vi "Begin.vi"(8 "error in":errorcluster) -> (0 "error out":errorcluster)   [LabVIEW 2015]
doc: "Called before other user functions, this VI is expected to open initial I/O refnums, load in file data, and do all program initialization. Notice that the <B>error out</B> terminal is simply used for data flow. Wiring it to other structures or subVIs ensures that this VI runs first."
uses:
  <vilib>/Rock Robotics/WPI/DriverStation/WPI_DriverStationRobotMode2.ctl
  <vilib>/Rock Robotics/WPI/Joystick/WPI_JoystickDeviceEnum.ctl
  <vilib>/Rock Robotics/SystemInterfaces/spilib/spi_bus.ctl
  <vilib>/Rock Robotics/WPI/CAN/TalonSRX/WPI_CANTalonSRX_APIControlMode.ctl
  <vilib>/Rock Robotics/WPI/CAN/TalonSRX/WPI_CANTalonSRX_APIFeedbackSelect.ctl
  <vilib>/Rock Robotics/SystemInterfaces/DIO/FPGA_DIOPWMChannel.ctl
  <vilib>/Rock Robotics/WPI/Solenoid/WPI_SolenoidChannel.ctl
  Robot Global Data.vi
  <vilib>/Rock Robotics/WPI/MotorControl/WPI_MotorControlOpenCANTalonSRX.vi
  <vilib>/Rock Robotics/WPI/Gyro/WPI_GyroXRS450_SPI_Open.vi
  <vilib>/Rock Robotics/WPI/Utilities/WPI_GetSetVariantRefNum.vi
  <vilib>/Rock Robotics/WPI/MotorControl/WPI_MotorControlOpen Talon.vi
  <vilib>/Rock Robotics/WPI/Solenoid/WPI_SolenoidOpenSingle.vi
  <vilib>/Rock Robotics/WPI/Solenoid/WPI_SolenoidOpenDouble.vi
  <vilib>/Rock Robotics/WPI/Counter/WPI_CounterDigitalInputToDigitalSource.vi
  <vilib>/Rock Robotics/SystemInterfaces/DIO/FPGA_DIOChannel.ctl
  <vilib>/Rock Robotics/WPI/Encoder/WPI_EncoderType.ctl
  <vilib>/Rock Robotics/SystemInterfaces/AI/FPGA_AIChannel.ctl
  <vilib>/Rock Robotics/WPI/Ultrasonic/WPI_SonarMB1010AnalogRefNum Registry Set.vi
  <vilib>/Rock Robotics/WPI/Ultrasonic/WPI_SonarMB1010AnalogOpen.vi
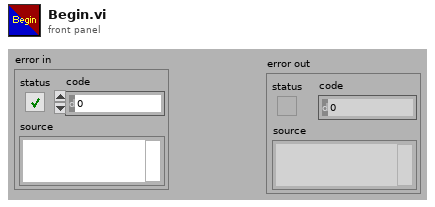
[diagram p1: front panel]
types:
  T1 = typedef "WPI_CANTalonSRX_APIFeedbackSelect.ctl" = enum16{"Digital Quadrature Encoder", "Analog Potentiometer", "Analog Encoder", "Count on Quad-A (Rising-Edge)", "Count on Quad-A (Falling-Edge)", "CTR Magnetic Enc (Absolute)", "CTR Magnetic Enc (Relative)", "Pulse Width"}
  T2 = typedef "FPGA_DIOPWMChannel.ctl" = enum8{"PWM 0", "PWM 1", "PWM 2", "PWM 3", "PWM 4", "PWM 5", "PWM 6", "PWM 7", "PWM 8", "PWM 9", "PWM MXP 0", "PWM MXP 1", "PWM MXP 2", "PWM MXP 3", "PWM MXP 4", "PWM MXP 5", "PWM MXP 6", "PWM MXP 7", "PWM MXP 8", "PWM MXP 9", "Invalid"}
  T3 = typedef "WPI_JoystickDeviceEnum.ctl" = enum16{"USB 0", "USB 1", "USB 2", "USB 3", "USB 4", "USB 5"}
  T4 = typedef "WPI_CANTalonSRX_APIControlMode.ctl" = enum8{"Percent VBus", "Speed", "Position", "Slave", "Unchanged / Invalid", "Voltage Compensation", "Current", "Motion Profile"}
  T5 = typedef "spi_bus.ctl" = enum16{"SPI On-Board, CS0", "SPI On-Board, CS1", "SPI On-Board, CS2", "SPI On-Board, CS3", "SPI MXP", "Invalid"}
  T6 = typedef "WPI_DriverStationRobotMode2.ctl" = enum16{"Autonomous Disabled", "Autonomous Enabled", "Teleop Disabled", "Teleop Enabled", "Disconnected", "Finish", "Test Disabled", "Test Enabled", "Emergency Stopped"}
  T7 = typedef "FPGA_AIChannel.ctl" = enum8{"AI 0", "AI 1", "AI 2", "AI 3", "AI MXP 0", "AI MXP 1", "AI MXP 2", "AI MXP 3", "Invalid"}
  T8 = typedef "WPI_SonarMB1010AnalogDeviceRef.ctl" = cluster{"AIDeviceRef":T9, "Scaling factor (V/in)":dbl, "Average Bits":u8}
  T9 = typedef "WPI_AnalogChannelDevRef.ctl" = cluster{"DevStatus":errorcluster, "Analog Channel":T7}
  T10 = typedef "WPI_SolenoidChannel.ctl" = enum8{"Solenoid 0", "Solenoid 1", "Solenoid 2", "Solenoid 3", "Solenoid 4", "Solenoid 5", "Solenoid 6", "Solenoid 7", "Invalid"}
  T11 = typedef "WPI_ServoDeviceRef.ctl" = cluster{"DeviceStatus":errorcluster, "PWM Channel":T2, "DeadBand":T12}
  T12 = typedef "WPI_PWMDeadband.ctl" = cluster{"Name":string, "maxPositivePwm":i32, "minPositivePwm":i32, "centerPwm":i32, "maxNegativePwm":i32, "minNegativePwm":i32, "angularRange":u16}
  T13 = typedef "WPI_SolenoidDevRef.ctl" = cluster{"DevStatus":errorcluster, "Pneumatics Control Module":u8, "Forward Solenoid Channel":T10, "Reverse Solenoid Channel":T10}
  T14 = typedef "WPI_MotorControlDeviceRef.ctl" = cluster{"DeviceStatus":errorcluster, "Type":T15, "PWM":cluster{"PWM Channel":T2, "DeadBand":T12}, "CAN":cluster{"Device Number":u8, "Control Mode":T16, "Semaphore":T17, "Max Vout":dbl, "TalonSRX Control Mode":T4}, "Invert":bool}
  T15 = typedef "WPI_MotorControlType.ctl" = enum16{"PWM", "CAN", "CANTalonSRX"}
  T16 = typedef "WPI_CANJaguar_ControlMode.ctl" = enum8{"Percent VBus", "Current", "Speed", "Position", "Voltage"}
  T17 = typedef "Semaphore RefNum" = refnum<k1>
  T18 = typedef "WPI_JoystickDevRef.ctl" = cluster{"Device":T3}
  T19 = typedef "WPI_GyroDevRef.ctl" = cluster{"DevStatus":errorcluster, "Analog Channel":T7, "Offset":dbl, "Gain (VoltsPerDegree/Second)":dbl, "Gyro Type":enum16{"Analog", "XRS450"}, "Handle":i32, "SPI Bus":T5, "Device Found":bool, "Sample Rate":dbl, "Calibrate On Open":bool}
  T20 = typedef "WPI_PotentiometerDevRef.ctl" = cluster{"DevStatus":errorcluster, "Analog Channel":T7, "Invert Output":bool}
  T21 = typedef "WPI_CompressorDevRef.ctl" = cluster{"DevStatus":errorcluster, "Pneumatics Control Module":u8}
  T22 = typedef "WPI_EncoderType.ctl" = enum16{"1x", "2x", "4x"}
  T23 = typedef "FPGA_DIOChannel.ctl" = enum8{"DIO 0", "DIO 1", "DIO 2", "DIO 3", "DIO 4", "DIO 5", "DIO 6", "DIO 7", "DIO 8", "DIO 9", "DIO MXP 0", "DIO MXP 1", "DIO MXP 2", "DIO MXP 3", "DIO MXP 4", "DIO MXP 5", "DIO MXP 6", "DIO MXP 7", "DIO MXP 8", "DIO MXP 9", "DIO MXP 10", "DIO MXP 11", "DIO MXP 12", "DIO MXP 13", "DIO MXP 14", "DIO MXP 15", "Invalid"}
  T24 = typedef "WPI_DigitalInputDevRef.ctl" = cluster{"DevStatus":errorcluster, "DIO Channel":T23}
  T25 = typedef "FPGA_CounterEncoderSourceConvertionLVSourceType.ctl" = cluster{"DevStatus":errorcluster, "AnalogTriggerMode?":bool, "DigitalMode":cluster{"DIO Channel":T26}, "AnalogTriggerMode":cluster{"AnalogTriggerIndex":T27, "OutputType":T28}}
  T26 = typedef "FPGA_DIODigitalSourceChannel.ctl" = enum8{"DIO 0", "DIO 1", "DIO 2", "DIO 3", "DIO 4", "DIO 5", "DIO 6", "DIO 7", "DIO 8", "DIO 9", "DIO MXP 0", "DIO MXP 1", "DIO MXP 2", "DIO MXP 3", "DIO MXP 4", "DIO MXP 5", "DIO MXP 6", "DIO MXP 7", "DIO MXP 8", "DIO MXP 9", "DIO MXP 10", "DIO MXP 11", "DIO MXP 12", "DIO MXP 13", "DIO MXP 14", "DIO MXP 15", "Disabled"}
  T27 = typedef "FPGA_AnalogTriggerIndex.ctl" = enum8{"Trig 0", "Trig 1", "Trig 2", "Trig 3", "Trig 4", "Trig 5", "Trig 6", "Trig 7", "Invalid"}
  T28 = typedef "FPGA_AnalogTriggerOutType.ctl" = enum16{"InWindow", "TriggerState", "Rising", "Falling"}
  T29 = typedef "WPI_EncoderDevRef.ctl" = cluster{"DevStatus":errorcluster, "EncoderIndex":T30, "CounterIndex":T31, "DistancePerCount":dbl, "Decoding Type":T22}
  T30 = typedef "FPGA_EncoderIdx.ctl" = enum8{"Enc 0", "Enc 1", "Enc 2", "Enc 3", "Enc 4", "Enc 5", "Enc 6", "Enc 7", "Invalid"}
  T31 = typedef "FPGA_CounterCtrSystemIndex.ctl" = enum8{"Ctr 0", "Ctr 1", "Ctr 2", "Ctr 3", "Ctr 4", "Ctr 5", "Ctr 6", "Ctr 7", "Invalid"}
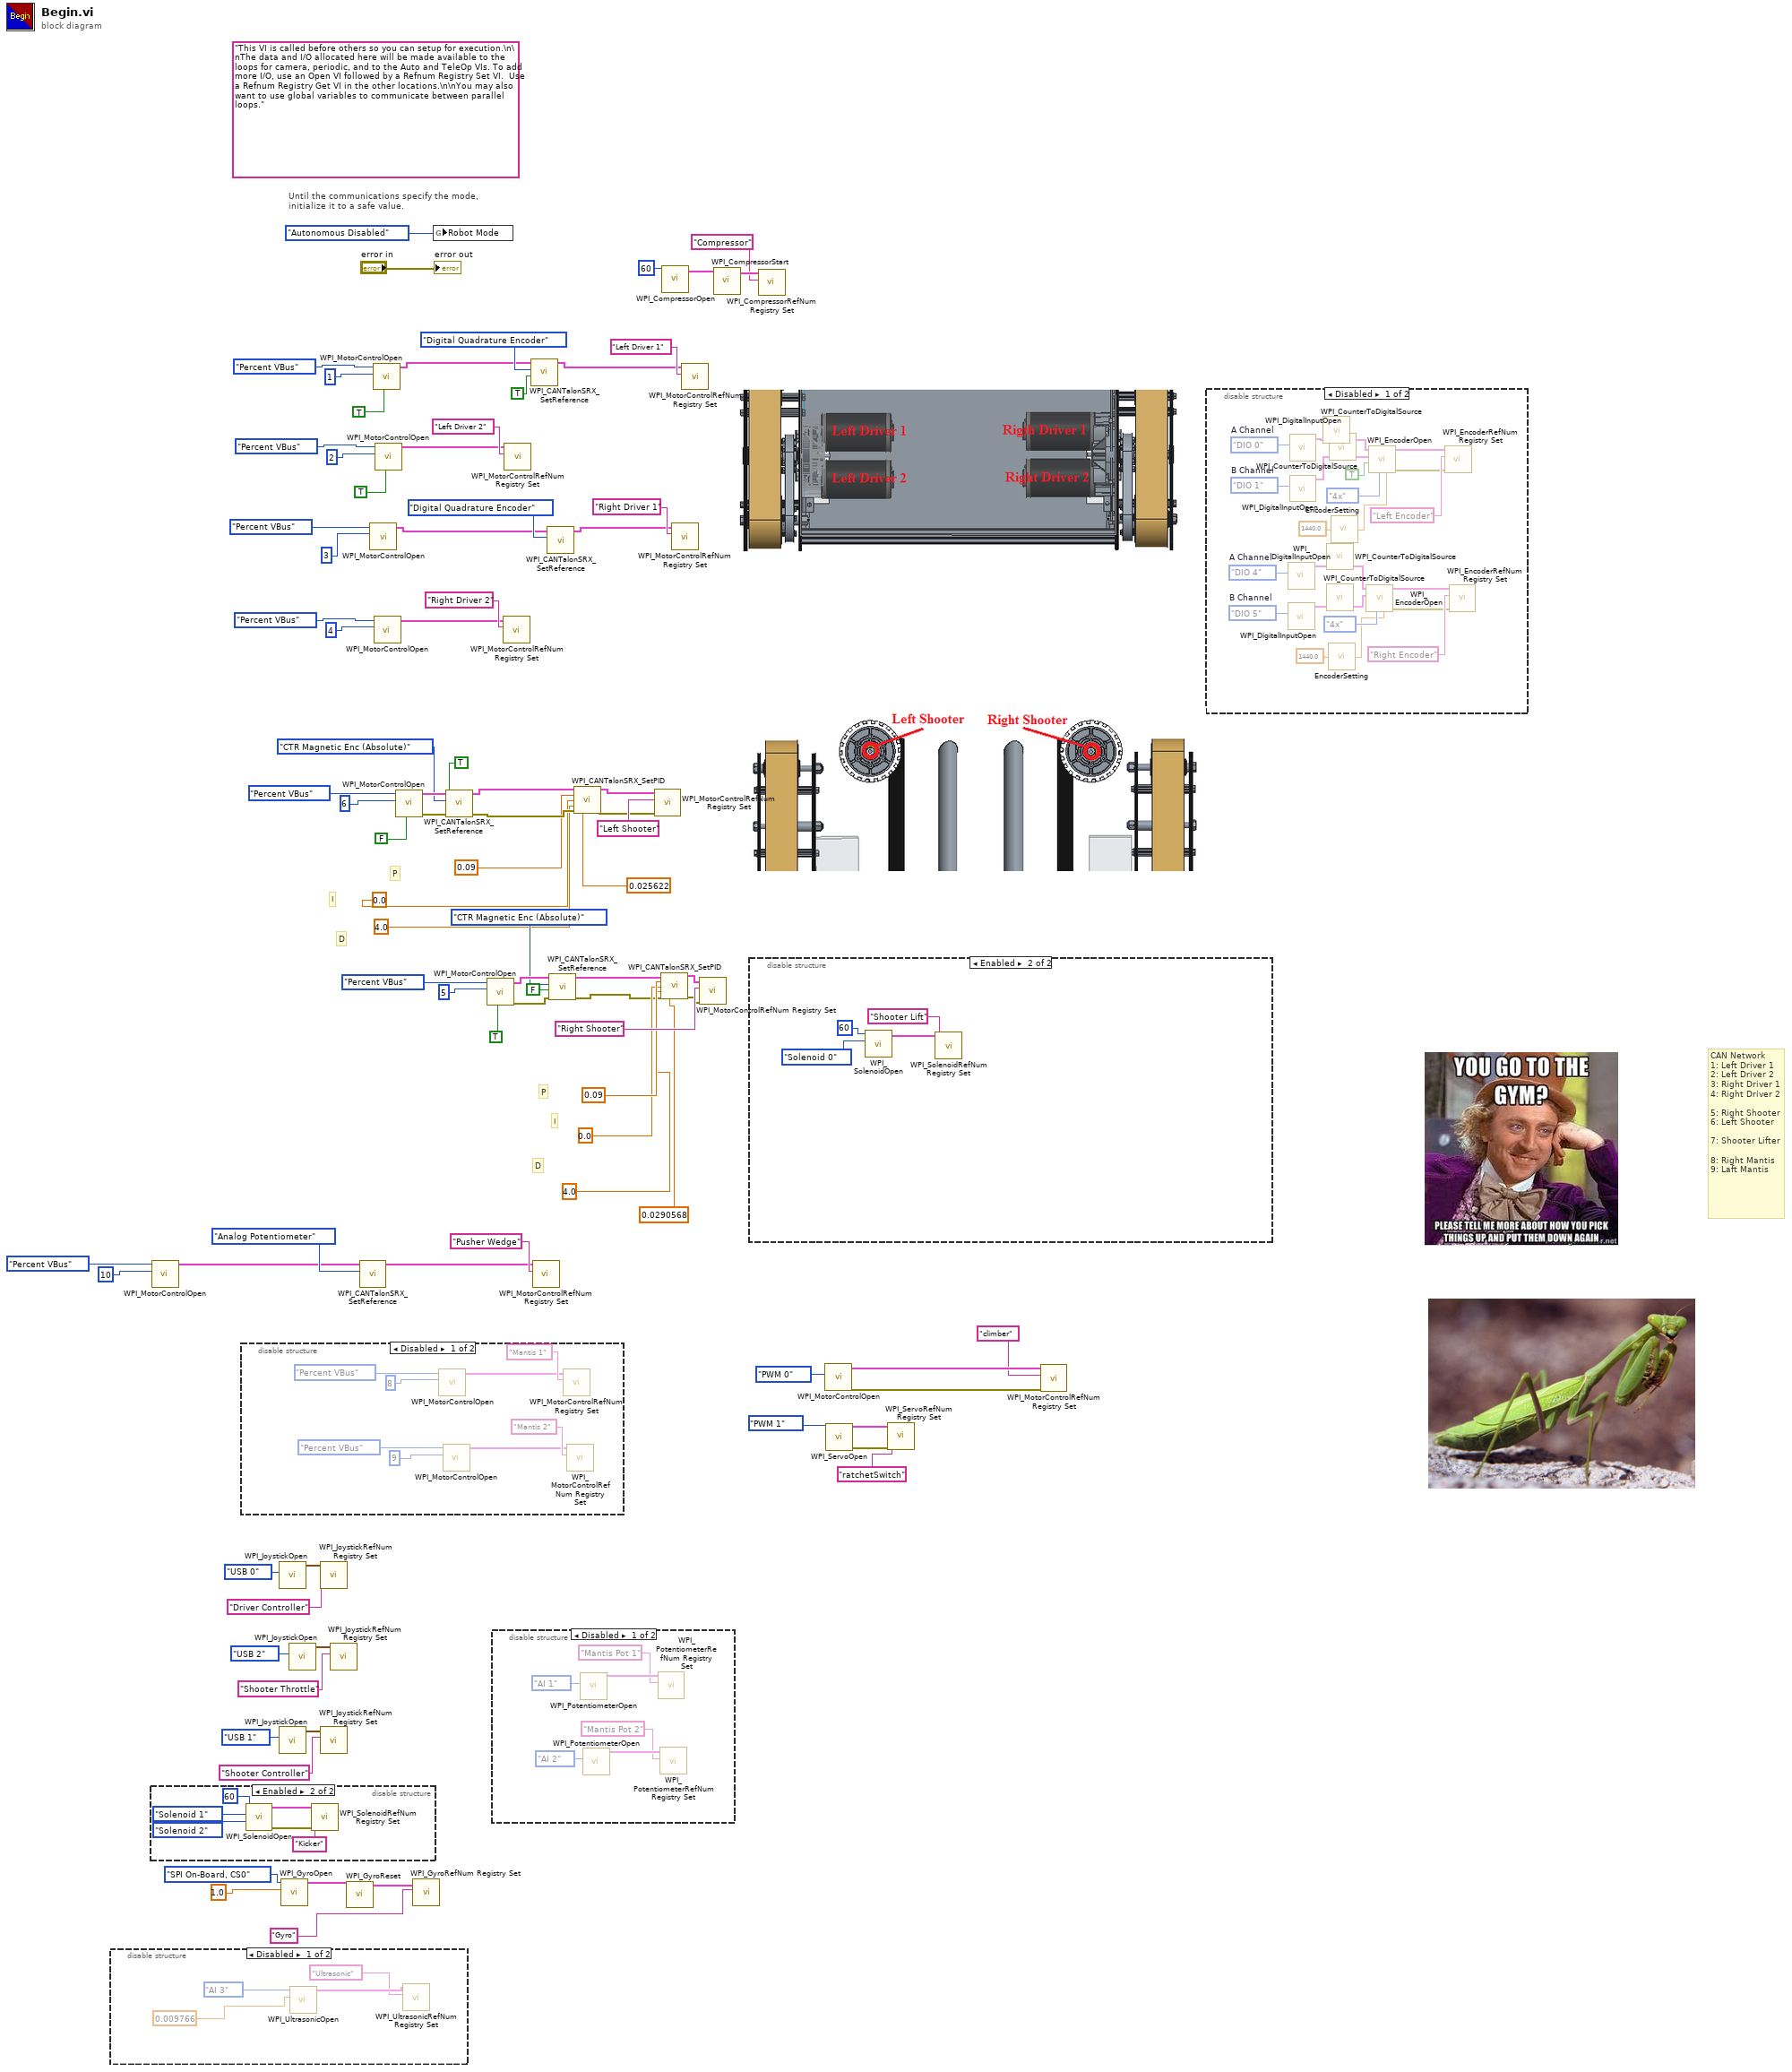
[diagram p0: block diagram]
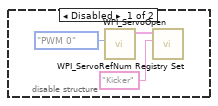
[diagram p3: hidden frame]
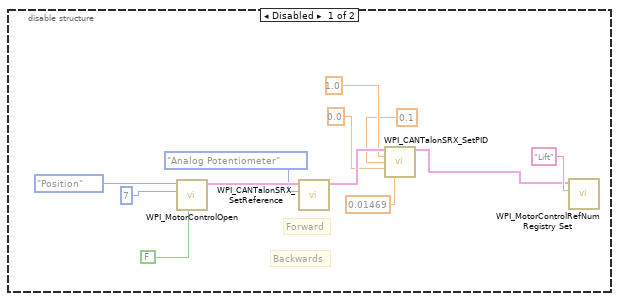
[diagram p4: hidden frame]
diagram:
  (unwired) "This VI is called before others so you can setup for execution.\n\nThe data and I/O allocated here will be made available to the loops for camera, periodic, and to the Auto and TeleOp VIs. To add more I/O, use an Open VI followed by a Refnum Registry Set VI.  Use a Refnum Registry Get VI in the other locations.\n\nYou may also want to use global variables to communicate between parallel loops."
  # "D"
  # "I"
  # "P"
  # "D"
  # "I"
  # "P"
  # "CAN Network\n1: Left Driver 1\n2: Left Driver 2\n3: Right Driver 1\n4: Right Driver 2\n\n5: Right Shooter\n6: Left Shooter\n\n7: Shooter Lifter\n\n8: Right Mantis\n9: Laft Mantis"
  # "Until the communications specify the mode,\ninitialize it to a safe value."
  n1 = disable-structure shown="Disabled" {
    frame Disabled {
      n2 = call-poly <vilib>:"WPI_UltrasonicOpen.vi"("Scaling factor (V/in)"=0.009766, "Analog Channel"=FPGA_AIChannel."AI 3") -> ("SonarMB1010AnalogDevRef"=w92:T8)  [unwired: 8 in, 1 out]
      n3 = call-poly <vilib>:"WPI_UltrasonicRefNum Registry Set.vi"("refnum name"="Ultrasonic", "SonarMB1010AnalogDevRef"=w92) -> ()  [unwired: 8 in, 2 out]
    }
    frame Enabled {
    }
  }
  n4 = disable-structure shown="Enabled" {
    frame Disabled {
      n5 = call <vilib>:"WPI_ServoOpen.vi"("PWM Channel"=FPGA_DIOPWMChannel."PWM 0") -> ("ServoDeviceRef"=w95:T11)  [unwired: 9 in, 1 out]
      n6 = call <vilib>:"WPI_ServoRefNum Registry Set.vi"("refnum name"="Kicker", "ServoDeviceRef"=w95) -> ()  [unwired: 8 in, 2 out]
    }
    frame Enabled {
      n7 = call-poly <vilib>:"WPI_SolenoidOpen.vi"("Reverse Solenoid Channel"=WPI_SolenoidChannel."Solenoid 2", "Forward Solenoid Channel"=WPI_SolenoidChannel."Solenoid 1", "Pneumatics Control Module (0)"=u8 60) -> ("error out"=w99:errorcluster, "SolenoidDevRef"=w100:T13)  [unwired: 7 in]
      n8 = call <vilib>:"WPI_SolenoidRefNum Registry Set.vi"("error in (no error)"=w99, "refnum name"="Kicker", "SolenoidDevRef"=w100) -> ()  [unwired: 7 in, 2 out]
    }
  }
  n9 = call-poly <vilib>:"WPI_MotorControlOpen.vi"("Device Number"=u8 10, "Control Mode"=WPI_CANTalonSRX_APIControlMode."Percent VBus") -> ("MotorControlDeviceRef"=w33:T14)  [unwired: 8 in, 1 out]
  n10 = disable-structure shown="Disabled" {
    frame Disabled {
      n11 = call-poly <vilib>:"WPI_MotorControlOpen.vi"("Device Number"=u8 8, "Control Mode"=WPI_CANTalonSRX_APIControlMode."Percent VBus") -> ("MotorControlDeviceRef"=w104:T14)  [unwired: 8 in, 1 out]
      n12 = call-poly <vilib>:"WPI_MotorControlOpen.vi"("Device Number"=u8 9, "Control Mode"=WPI_CANTalonSRX_APIControlMode."Percent VBus") -> ("MotorControlDeviceRef"=w103:T14)  [unwired: 8 in, 1 out]
      n13 = call <vilib>:"WPI_MotorControlRefNum Registry Set.vi"("refnum name"="Mantis 1", "MotorControlDevRef"=w104) -> ()  [unwired: 8 in, 2 out]
      n14 = call <vilib>:"WPI_MotorControlRefNum Registry Set.vi"("refnum name"="Mantis 2", "MotorControlDevRef"=w103) -> ()  [unwired: 8 in, 2 out]
    }
    frame Enabled {
    }
  }
  n15 = call <vilib>:"WPI_JoystickOpen.vi"("JoystickDevice"=WPI_JoystickDeviceEnum."USB 0") -> ("JoystickDevRef"=w70:T18)  [unwired: 10 in]
  n16 = call <vilib>:"WPI_JoystickOpen.vi"("JoystickDevice"=WPI_JoystickDeviceEnum."USB 1") -> ("JoystickDevRef"=w71:T18)  [unwired: 10 in]
  n17 = call-poly <vilib>:"WPI_GyroOpen.vi"("Sample Rate (ms)"=1.0, "SPI Bus"=spi_bus."SPI On-Board, CS0") -> ("GyroDevRef"=w65:T19)  [unwired: 8 in, 1 out]
  n18 = call <vilib>:"WPI_JoystickOpen.vi"("JoystickDevice"=WPI_JoystickDeviceEnum."USB 2") -> ("JoystickDevRef"=w31:T18)  [unwired: 10 in]
  n19 = call <vilib>:"WPI_JoystickRefNum Registry Set.vi"("refnum name"="Driver Controller", "JoystickDevRef"=w70) -> ()  [unwired: 8 in, 2 out]
  n20 = call <vilib>:"WPI_JoystickRefNum Registry Set.vi"("refnum name"="Shooter Controller", "JoystickDevRef"=w71) -> ()  [unwired: 8 in, 2 out]
  n21 = call <vilib>:"WPI_JoystickRefNum Registry Set.vi"("refnum name"="Shooter Throttle", "JoystickDevRef"=w31) -> ()  [unwired: 8 in, 2 out]
  n22 = call <vilib>:"WPI_GyroReset.vi"("GyroDevRef"=w65) -> ("GyroDevRef"=w64:T19)  [unwired: 9 in, 1 out]
  n23 = call <vilib>:"WPI_CANTalonSRX_SetReference.vi"("Feedback Reference"=WPI_CANTalonSRX_APIFeedbackSelect."Analog Potentiometer", "CAN Talon SRX Ref"=w33) -> ("CAN Talon SRX Ref"=w25:T14)  [unwired: 8 in, 1 out]
  n24 = call-poly <vilib>:"WPI_MotorControlOpen.vi"("Device Number"=u8 3, "Control Mode"=WPI_CANTalonSRX_APIControlMode."Percent VBus") -> ("MotorControlDeviceRef"=w6:T14)  [unwired: 8 in, 1 out]
  n25 = call-poly <vilib>:"WPI_MotorControlOpen.vi"("Invert"=TRUE, "Device Number"=u8 1, "Control Mode"=WPI_CANTalonSRX_APIControlMode."Percent VBus") -> ("MotorControlDeviceRef"=w3:T14)  [unwired: 7 in, 1 out]
  n26 = call-poly <vilib>:"WPI_MotorControlOpen.vi"("Device Number"=u8 4, "Control Mode"=WPI_CANTalonSRX_APIControlMode."Percent VBus") -> ("MotorControlDeviceRef"=w20:T14)  [unwired: 8 in, 1 out]
  n27 = call-poly <vilib>:"WPI_MotorControlOpen.vi"("Invert"=TRUE, "Device Number"=u8 2, "Control Mode"=WPI_CANTalonSRX_APIControlMode."Percent VBus") -> ("MotorControlDeviceRef"=w19:T14)  [unwired: 7 in, 1 out]
  n28 = call-poly <vilib>:"WPI_MotorControlOpen.vi"("Invert"=FALSE, "Device Number"=u8 6, "Control Mode"=WPI_CANTalonSRX_APIControlMode."Percent VBus") -> ("error out"=w53:errorcluster, "MotorControlDeviceRef"=w52:T14)  [unwired: 7 in]
  n29 = call <vilib>:"WPI_GyroRefNum Registry Set.vi"("refnum name"="Gyro", "GyroDevRef"=w64) -> ()  [unwired: 8 in, 2 out]
  n30 = global write "Robot Global Data.vi" "Robot Mode"(WPI_DriverStationRobotMode2."Autonomous Disabled" ("Robot Mode")) -> ()
  n31 = call <vilib>:"WPI_CANTalonSRX_SetReference.vi"("error in (no error)"=w53, "Reverse Feedback Sensor"=TRUE, "Feedback Reference"=WPI_CANTalonSRX_APIFeedbackSelect."CTR Magnetic Enc (Absolute)", "CAN Talon SRX Ref"=w52) -> ("error out"=w47:errorcluster, "CAN Talon SRX Ref"=w24:T14)  [unwired: 6 in]
  n32 = call-poly <vilib>:"WPI_MotorControlOpen.vi"("Invert"=TRUE, "Device Number"=u8 5, "Control Mode"=WPI_CANTalonSRX_APIControlMode."Percent VBus") -> ("error out"=w49:errorcluster, "MotorControlDeviceRef"=w50:T14)  [unwired: 7 in]
  n33 = disable-structure shown="Disabled" {
    frame Disabled {
      n34 = call <vilib>:"WPI_PotentiometerOpen.vi"("Analog Channel"=FPGA_AIChannel."AI 1") -> ("PotDevRef"=w115:T20)  [unwired: 9 in, 1 out]
      n35 = call <vilib>:"WPI_PotentiometerOpen.vi"("Analog Channel"=FPGA_AIChannel."AI 2") -> ("PotDevRef"=w112:T20)  [unwired: 9 in, 1 out]
      n36 = call <vilib>:"WPI_PotentiometerRefNum Registry Set.vi"("refnum name"="Mantis Pot 1", "PotDevRef"=w115) -> ()  [unwired: 8 in, 2 out]
      n37 = call <vilib>:"WPI_PotentiometerRefNum Registry Set.vi"("refnum name"="Mantis Pot 2", "PotDevRef"=w112) -> ()  [unwired: 8 in, 2 out]
    }
    frame Enabled {
    }
  }
  n38 = call <vilib>:"WPI_MotorControlRefNum Registry Set.vi"("refnum name"="Right Driver 2", "MotorControlDevRef"=w20) -> ()  [unwired: 8 in, 2 out]
  n39 = call <vilib>:"WPI_MotorControlRefNum Registry Set.vi"("refnum name"="Left Driver 2", "MotorControlDevRef"=w19) -> ()  [unwired: 8 in, 2 out]
  n40 = call <vilib>:"WPI_CANTalonSRX_SetReference.vi"("Reverse Feedback Sensor"=TRUE, "Feedback Reference"=WPI_CANTalonSRX_APIFeedbackSelect."Digital Quadrature Encoder", "CAN Talon SRX Ref"=w3) -> ("CAN Talon SRX Ref"=w2:T14)  [unwired: 7 in, 1 out]
  n41 = call <vilib>:"WPI_MotorControlRefNum Registry Set.vi"("refnum name"="Pusher Wedge", "MotorControlDevRef"=w25) -> ()  [unwired: 8 in, 2 out]
  n42 = call <vilib>:"WPI_CANTalonSRX_SetReference.vi"("Feedback Reference"=WPI_CANTalonSRX_APIFeedbackSelect."Digital Quadrature Encoder", "CAN Talon SRX Ref"=w6) -> ("CAN Talon SRX Ref"=w5:T14)  [unwired: 8 in, 1 out]
  n43 = call <vilib>:"WPI_CANTalonSRX_SetReference.vi"("error in (no error)"=w49, "Reverse Feedback Sensor"=FALSE, "Feedback Reference"=WPI_CANTalonSRX_APIFeedbackSelect."CTR Magnetic Enc (Absolute)", "CAN Talon SRX Ref"=w50) -> ("error out"=w22:errorcluster, "CAN Talon SRX Ref"=w23:T14)  [unwired: 6 in]
  n44 = call <vilib>:"WPI_CANTalonSRX_SetPID.vi"("CAN Talon SRX Ref"=w24, "P"=0.09 ("P Left"), "I"=0.0 ("I Left"), "D"=4.0 ("D left"), "error in (no error)"=w47, "F"=0.025622 ("F left")) -> ("CAN Talon SRX Ref"=w36:T14, "error out"=w35:errorcluster)  [unwired: 8 in]
  n45 = call <vilib>:"WPI_MotorControlRefNum Registry Set.vi"("error in (no error)"=w35, "refnum name"="Left Shooter", "MotorControlDevRef"=w36) -> ()  [unwired: 7 in, 2 out]
  n46 = call <vilib>:"WPI_CANTalonSRX_SetPID.vi"("CAN Talon SRX Ref"=w23, "P"=0.09 ("P Right"), "I"=0.0 ("I right"), "D"=4.0 ("d right"), "error in (no error)"=w22, "F"=0.0290568 ("F right")) -> ("CAN Talon SRX Ref"=w46:T14, "error out"=w45:errorcluster)  [unwired: 8 in]
  n47 = call <vilib>:"WPI_CompressorOpen.vi"("Pneumatics Control Module (0)"=u8 60) -> ("CompressorDevRef"=w28:T21)  [unwired: 13 in, 1 out]
  n48 = call <vilib>:"WPI_MotorControlRefNum Registry Set.vi"("refnum name"="Right Driver 1", "MotorControlDevRef"=w5) -> ()  [unwired: 8 in, 2 out]
  n49 = call <vilib>:"WPI_MotorControlRefNum Registry Set.vi"("refnum name"="Left Driver 1", "MotorControlDevRef"=w2) -> ()  [unwired: 8 in, 2 out]
  n50 = call <vilib>:"WPI_MotorControlRefNum Registry Set.vi"("error in (no error)"=w45, "refnum name"="Right Shooter", "MotorControlDevRef"=w46) -> ()  [unwired: 7 in, 2 out]
  n51 = call <vilib>:"WPI_CompressorStart.vi"("CompressorDevRef"=w28) -> ("CompressorDevRef"=w27:T21)  [unwired: 9 in, 1 out]
  n52 = disable-structure shown="Enabled" {
    frame Disabled {
      # "Backwards"
      # "Forward"
      n53 = call-poly <vilib>:"WPI_MotorControlOpen.vi"("Invert"=FALSE, "Device Number"=u8 7, "Control Mode"=WPI_CANTalonSRX_APIControlMode."Position") -> ("MotorControlDeviceRef"=w125:T14)  [unwired: 7 in, 1 out]
      n54 = call <vilib>:"WPI_CANTalonSRX_SetReference.vi"("Feedback Reference"=WPI_CANTalonSRX_APIFeedbackSelect."Analog Potentiometer", "CAN Talon SRX Ref"=w125) -> ("CAN Talon SRX Ref"=w123:T14)  [unwired: 8 in, 1 out]
      n55 = call <vilib>:"WPI_CANTalonSRX_SetPID.vi"("CAN Talon SRX Ref"=w123, "P"=1.0 ("P Right"), "I"=0.1 ("d right"), "D"=0.0 ("I right"), "F"=0.01469) -> ("CAN Talon SRX Ref"=w118:T14)  [unwired: 9 in, 1 out]
      n56 = call <vilib>:"WPI_MotorControlRefNum Registry Set.vi"("refnum name"="Lift", "MotorControlDevRef"=w118) -> ()  [unwired: 8 in, 2 out]
    }
    frame Enabled {
      n57 = call-poly <vilib>:"WPI_SolenoidOpen.vi"("Solenoid Channel"=WPI_SolenoidChannel."Solenoid 0", "Pneumatics Control Module (0)"=u8 60) -> ("SolenoidDevRef"=w132:T13)  [unwired: 8 in, 1 out]
      n58 = call <vilib>:"WPI_SolenoidRefNum Registry Set.vi"("refnum name"="Shooter Lift", "SolenoidDevRef"=w132) -> ()  [unwired: 8 in, 2 out]
    }
  }
  n59 = call <vilib>:"WPI_CompressorRefNum Registry Set.vi"("refnum name"="Compressor", "CompressorDevRef"=w27) -> ()  [unwired: 8 in, 2 out]
  n60 = call-poly <vilib>:"WPI_MotorControlOpen.vi"("PWM Channel"=FPGA_DIOPWMChannel."PWM 0") -> ("error out"=w12:errorcluster, "MotorControlDeviceRef"=w14:T14)  [unwired: 9 in]
  n61 = call <vilib>:"WPI_ServoOpen.vi"("PWM Channel"=FPGA_DIOPWMChannel."PWM 1") -> ("error out"=w9:errorcluster, "ServoDeviceRef"=w10:T11)  [unwired: 9 in]
  n62 = call <vilib>:"WPI_ServoRefNum Registry Set.vi"("error in (no error)"=w9, "refnum name"="ratchetSwitch", "ServoDeviceRef"=w10) -> ()  [unwired: 7 in, 2 out]
  n63 = call <vilib>:"WPI_MotorControlRefNum Registry Set.vi"("error in (no error)"=w12, "refnum name"="climber", "MotorControlDevRef"=w14) -> ()  [unwired: 7 in, 2 out]
  n64 = disable-structure shown="Disabled" {
    frame Disabled {
      w151 = FPGA_DIOChannel."DIO 5"  # B Channel
      w150 = FPGA_DIOChannel."DIO 4"  # A Channel
      w157 = FPGA_DIOChannel."DIO 1"  # B Channel
      w156 = FPGA_DIOChannel."DIO 0"  # A Channel
      n65 = call <vilib>:"WPI_DigitalInputOpen.vi"("DIO Channel"=w150) -> ("DigitalInputDevRef"=w147:T24)  [unwired: 1 in, 9 out]
      n66 = call <vilib>:"WPI_DigitalInputOpen.vi"("DIO Channel"=w151) -> ("DigitalInputDevRef"=w148:T24)  [unwired: 1 in, 9 out]
      n67 = call <vilib>:"WPI_DigitalInputOpen.vi"("DIO Channel"=w156) -> ("DigitalInputDevRef"=w153:T24)  [unwired: 1 in, 9 out]
      n68 = call <vilib>:"WPI_DigitalInputOpen.vi"("DIO Channel"=w157) -> ("DigitalInputDevRef"=w154:T24)  [unwired: 1 in, 9 out]
      n69 = call-poly <vilib>:"WPI_CounterToDigitalSource.vi"("DigitalInputDevRef"=w153) -> ("Digital Source"=w152:T25)  [unwired: 6 out]
      n70 = call-poly <vilib>:"WPI_CounterToDigitalSource.vi"("DigitalInputDevRef"=w147) -> ("Digital Source"=w146:T25)  [unwired: 6 out]
      n71 = call-poly <vilib>:"WPI_CounterToDigitalSource.vi"("DigitalInputDevRef"=w148) -> ("Digital Source"=w149:T25)  [unwired: 6 out]
      n72 = call "EncoderSetting.vi"("Line Count (Encoder)"=1440.0) -> ("DistancePerCount"=w139:dbl)
      n73 = call-poly <vilib>:"WPI_CounterToDigitalSource.vi"("DigitalInputDevRef"=w154) -> ("Digital Source"=w155:T25)  [unwired: 6 out]
      n74 = call "EncoderSetting.vi"("Line Count (Encoder)"=1440.0) -> ("DistancePerCount"=w140:dbl)
      n75 = call <vilib>:"WPI_EncoderOpen.vi"("DistancePerCount"=w139, "Decoding Type"=WPI_EncoderType."4x", "BSource"=w149, "ASource"=w146) -> ("error out"=w135:errorcluster, "EncoderDevRef"=w136:T29)  [unwired: 4 in, 2 out]
      n76 = call <vilib>:"WPI_EncoderOpen.vi"("DistancePerCount"=w140, "Decoding Type"=WPI_EncoderType."4x", "Invert Direction (False)"=TRUE, "BSource"=w155, "ASource"=w152) -> ("error out"=w133:errorcluster, "EncoderDevRef"=w134:T29)  [unwired: 3 in, 2 out]
      n77 = call <vilib>:"WPI_EncoderRefNum Registry Set.vi"("error in (no error)"=w133, "refnum name"="Left Encoder", "EncoderDevRef"=w134) -> ()  [unwired: 7 in, 2 out]
      n78 = call <vilib>:"WPI_EncoderRefNum Registry Set.vi"("error in (no error)"=w135, "refnum name"="Right Encoder", "EncoderDevRef"=w136) -> ()  [unwired: 7 in, 2 out]
    }
    frame Enabled {
    }
  }
  "error out" <- "error in"
